vi "WriteChecksum.vi"(8 "error in (no error)":errorcluster, 11 "CS++Message in":refnum<class "CS++Message.lvclass">) -> (0 "error out":errorcluster, 3 "CS++Message out":refnum<class "CS++Message.lvclass">)   [LabVIEW 2014, in "CS++Message.lvlib" / "CS++Message.lvclass"]
uses:
  CS++Message.lvclass
  CS++Message.lvclass/CS++Message.ctl
  <vilib>/Utility/traverseref.llb/TRef TravTarget.ctl
  <vilib>/Utility/traverseref.llb/VI Scripting - Traverse.lvlib
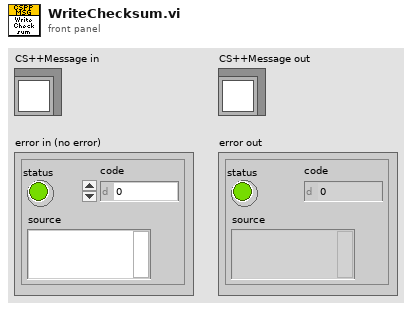
[diagram p1: front panel]
types:
  T1 = typedef "TRef TravTarget.ctl" = enum16{"FP", "BD", "Other"}
  T2 = typedef "imagedata.ctl" = cluster{"image type":i32, "image depth":i32, "image":u8[], "mask":u8[], "colors":u32[], "Rectangle":cluster{"left":i16, "top":i16, "right":i16, "bottom":i16}}
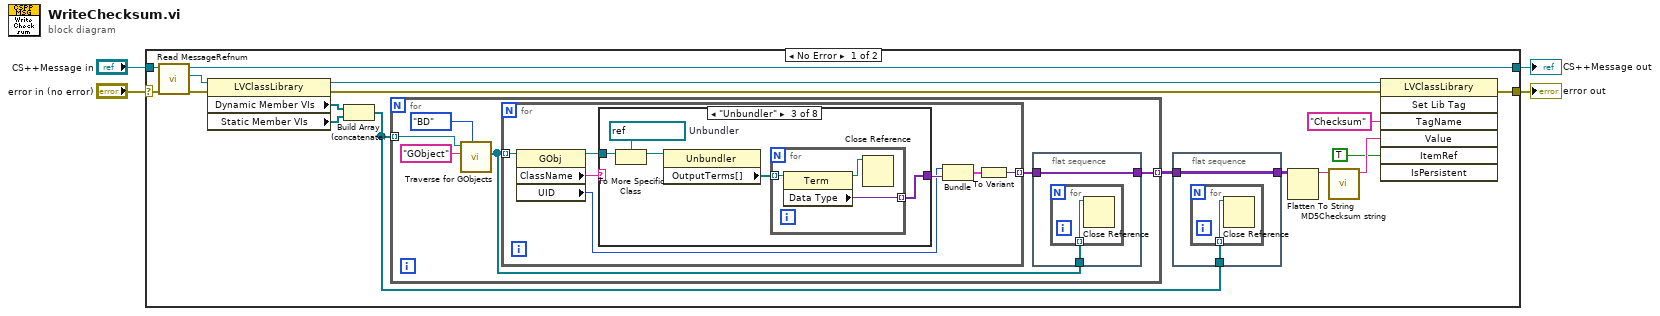
[diagram p0: block diagram]
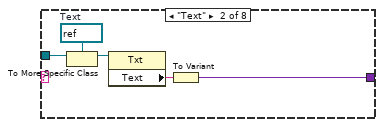
[diagram p3: hidden frame]
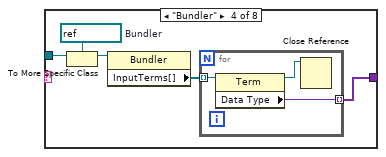
[diagram p4: hidden frame]
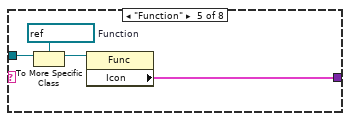
[diagram p5: hidden frame]
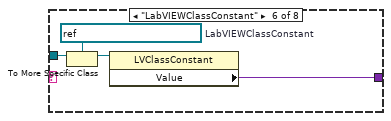
[diagram p6: hidden frame]
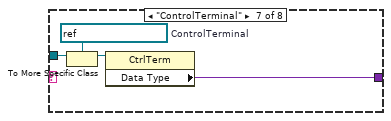
[diagram p7: hidden frame]
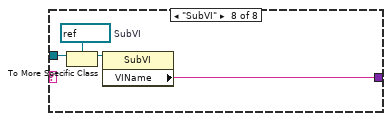
[diagram p8: hidden frame]
diagram:
  n1 = case shown="No Error" "error in (no error)" {
    selector: "error in (no error)" -> [w18 w79]
    tunnel: [w17 w79] -> w3
    tunnel: [w19 w78] -> w1
    tunnel: "CS++Message in" -> [w20 w78]
    frame No Error {
      n2 = call "Read MessageRefnum.vi"("error in (no error)"=w18, "CS++Message in"=w20) -> ("error out"=w8:errorcluster, "MessageRefnum"=w10:refnum<vi>, "CS++Message out"=w19:refnum<class "CS++Message.lvclass">)  [unwired: 7 in]
      n3 = property class="LVClassLibrary"(reference=w10, error in=w8) -> (reference out=w9:refnum<vi>, error out=w7:errorcluster, "Dynamic Member VIs"=w16:refnum<vi>[], "Static Member VIs"=w15:refnum<vi>[])
      n4 = Build Array (concatenate)(w16, w15) -> (w11:refnum<vi>[])
      n5 = for {
        tunnel: w11 -> [w28] mode=indexing
        tunnel: [w27] -> w13 mode=indexing
        n6 = call <vilib>:"Traverse for GObjects.vi"("Traverse Target"=TRef_TravTarget."BD", "Class Name"="GObject", "VI Refnum"=w28) -> ("References"=w25:refnum<vi>[])  [unwired: 5 in, 3 out]
        n7 = for {
          tunnel: w25 -> [w40] mode=indexing
          tunnel: [w34] -> w26 mode=indexing
          n8 = property class="GObj"(reference=w40) -> (reference out=w39:refnum<vi>, "ClassName"=w38:string, "UID"=w36:i32)  [unwired: 1 in, 1 out]
          n9 = case shown="\"Unbundler\"" w38 {
            tunnel: w39 -> [_ w44 w49 w57 w64 w68 w72 w76]
            tunnel: [_ w41 w46 w54 w62 w67 w70 w74] -> w37
            frame Default {
            }
            frame "Text" {
              w45 = refnum<vi> refnum  # Text
              n10 = To More Specific Class(target class=w45, reference=w44) -> (specific class reference=w43:refnum<vi>)  [unwired: 1 in, 1 out]
              n11 = property class="Txt"(reference=w43) -> ("Text"=w42:string)  [unwired: 1 in, 2 out]
              n12 = To Variant(anything=w42) -> (Variant=w41:variant)
            }
            frame "Unbundler" {
              w50 = refnum<vi> refnum  # Unbundler
              n13 = To More Specific Class(target class=w50, reference=w49) -> (specific class reference=w48:refnum<vi>)  [unwired: 1 in, 1 out]
              n14 = property class="Unbundler"(reference=w48) -> ("OutputTerms[]"=w47:refnum<vi>[])  [unwired: 1 in, 2 out]
              n15 = for {
                tunnel: w47 -> [w53] mode=indexing
                tunnel: [w52] -> w46 mode=indexing
                n16 = property class="Term"(reference=w53) -> (reference out=w51:refnum<vi>, "Data Type"=w52:variant)  [unwired: 1 in, 1 out]
                n17 = Close Reference(reference=w51) -> ()  [unwired: 1 in, 1 out]
              }
            }
            frame "Bundler" {
              w58 = refnum<vi> refnum  # Bundler
              n18 = To More Specific Class(target class=w58, reference=w57) -> (specific class reference=w56:refnum<vi>)  [unwired: 1 in, 1 out]
              n19 = property class="Bundler"(reference=w56) -> ("InputTerms[]"=w55:refnum<vi>[])  [unwired: 1 in, 2 out]
              n20 = for {
                tunnel: w55 -> [w61] mode=indexing
                tunnel: [w60] -> w54 mode=indexing
                n21 = property class="Term"(reference=w61) -> (reference out=w59:refnum<vi>, "Data Type"=w60:variant)  [unwired: 1 in, 1 out]
                n22 = Close Reference(reference=w59) -> ()  [unwired: 1 in, 1 out]
              }
            }
            frame "Function" {
              w65 = refnum<vi> refnum  # Function
              n23 = To More Specific Class(target class=w65, reference=w64) -> (specific class reference=w63:refnum<vi>)  [unwired: 1 in, 1 out]
              n24 = property class="Func"(reference=w63) -> ("Icon"=w62:T2)  [unwired: 1 in, 2 out]
            }
            frame "LabVIEWClassConstant" {
              w69 = refnum<vi> refnum  # LabVIEWClassConstant
              n25 = To More Specific Class(target class=w69, reference=w68) -> (specific class reference=w66:refnum<vi>)  [unwired: 1 in, 1 out]
              n26 = property class="LVClassConstant"(reference=w66) -> ("Value"=w67:variant)  [unwired: 1 in, 2 out]
            }
            frame "ControlTerminal" {
              w73 = refnum<vi> refnum  # ControlTerminal
              n27 = To More Specific Class(target class=w73, reference=w72) -> (specific class reference=w71:refnum<vi>)  [unwired: 1 in, 1 out]
              n28 = property class="CtrlTerm"(reference=w71) -> ("Data Type"=w70:variant)  [unwired: 1 in, 2 out]
            }
            frame "SubVI" {
              w77 = refnum<vi> refnum  # SubVI
              n29 = To More Specific Class(target class=w77, reference=w76) -> (specific class reference=w75:refnum<vi>)  [unwired: 1 in, 1 out]
              n30 = property class="SubVI"(reference=w75) -> ("VIName"=w74:string)  [unwired: 1 in, 2 out]
            }
          }
          n31 = Bundle("UID"=w36, "Data Type"=w37) -> (w35:cluster{"UID":i32, "Data Type":variant})  [unwired: 1 in]
          n32 = To Variant(anything=w35) -> (Variant=w34:variant)
        }
        n33 = flat-sequence {
          tunnel: [w32] -> w27
          tunnel: w26 -> [w32]
          tunnel: w25 -> [w31]
          frame #0 {
            n34 = for {
              tunnel: w31 -> [w33] mode=indexing
              n35 = Close Reference(reference=w33) -> ()  [unwired: 1 in, 1 out]
            }
          }
        }
      }
      n36 = flat-sequence {
        tunnel: w13 -> [w22]
        tunnel: w11 -> [w23]
        tunnel: [w22] -> w12
        frame #0 {
          n37 = for {
            tunnel: w23 -> [w24] mode=indexing
            n38 = Close Reference(reference=w24) -> ()  [unwired: 1 in, 1 out]
          }
        }
      }
      n39 = Flatten To String(anything=w12) -> (data string=w14:string)  [unwired: 3 in, 2 out]
      n40 = call <vilib>:"MD5Checksum string.vi"("Message String"=w14) -> ("MD5 message-digest"=w6:string)  [unwired: 10 in]
      n41 = invoke class="LVClassLibrary" method="Set Lib Tag"(reference=w9, error in=w7, "TagName"="Checksum" ("Tag Name"), "Value"=w6, "ItemRef"=TRUE ("Is Persistent")) -> (error out=w17:errorcluster)  [unwired: 2 in, 6 out]
    }
    frame Error {
    }
  }
  "error out" <- w3
  "CS++Message out" <- w1
